vi "rotation U16 img (SubVI).vi"(10 "oblique angle [deg]":dbl, 11 "Image Pixels (U16) in":u16[][](array[numeric])) -> (3 "Image Pixels (U16) out":u16[][](array[numeric]))   [LabVIEW 2024]
uses:
  <vilib>/vision/NI_Vision_Development_Module.lvlib
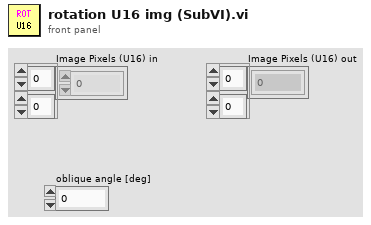
[diagram p1: front panel]
types:
  T1 = typedef "Image Type" = u32
  T2 = typedef "IMAQ Image.ctl" = refnum<image>
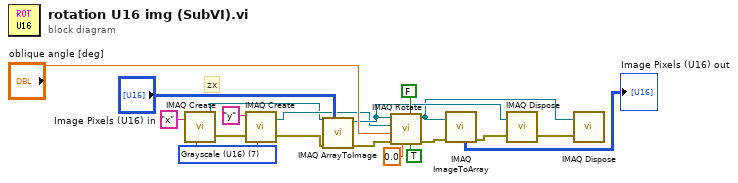
[diagram p0: block diagram]
diagram:
  w11 = T1 7 items=["Grayscale (U8)", "Grayscale (I16)", "Grayscale (SGL)", "Complex (CSG)", "RGB (U32)", "HSL (U32)", "RGB (U64)", "Grayscale (U16)"] ("Image Type")
  # "zx"
  n1 = call "IMAQ Create"("Image Name"="x", "Image Type"=w11) -> ("New Image"=w7:T2, "error out"=w1:errorcluster)  [unwired: 3 in]
  n2 = call "IMAQ Create"("Image Name"="y", "Image Type"=w11, "error in (no error)"=w1) -> ("New Image"=w13:T2, "error out"=w2:errorcluster)  [unwired: 2 in]
  n3 = call "IMAQ ArrayToImage"("Image Pixels (U16)"="Image Pixels (U16) in", "error in (no error)"=w2, "Image"=w7) -> ("error out"=w10:errorcluster, "Image Out"=w14:T2)  [unwired: 7 in]
  n4 = call "IMAQ Rotate"("Use Bilinear Interpolation"=TRUE, "Maintain Size"=FALSE, "Replace Value"=sgl 0.0, "error in (no error)"=w10, "Angle (degrees)"="oblique angle [deg]", "Image Dst"=w13, "Image Src"=w14) -> ("error out"=w8:errorcluster, "Image Dst Out"=w9:T2)  [unwired: 3 in]
  n5 = call "IMAQ ImageToArray"("error in (no error)"=w8, "Image"=w9) -> ("Image Pixels (U16)"=→"Image Pixels (U16) out":u16[][], "error out"=w3:errorcluster)  [unwired: 2 in, 3 out]
  n6 = call "IMAQ Dispose"("Image"=w14, "error in (no error)"=w3) -> ("error out"=w4:errorcluster)  [unwired: 4 in]
  n7 = call "IMAQ Dispose"("Image"=w9, "error in (no error)"=w4) -> ()  [unwired: 4 in, 1 out]
